vi "SAE J-1939 Gaslist add Signal Comments.vi"(10 "FTIR 1 Index":i32[](array[numeric])) -> (2 "FTIR 1 Name out":T1[](array[typedef]))   [LabVIEW 2020, in "CAN Konfig.lvlib"]
uses:
  CAN Konfig.lvlib
  Visualisierungs Elemente/String - Ausgabefeld.ctl
  FT-IR/FGV FT-IR Gasliste Aktionen.ctl
  <vilib>/regexp/Match Regular Expression.xnode
  FT-IR/FT-IR.lvlib
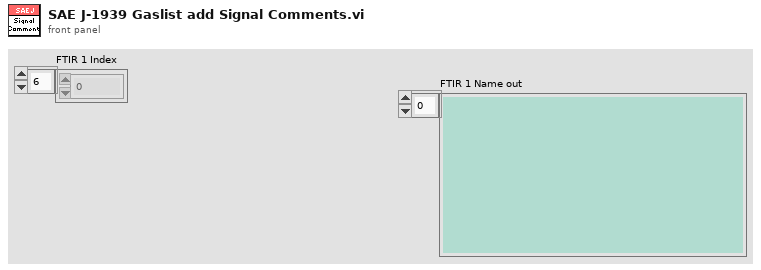
[diagram p1: front panel]
types:
  T1 = typedef "String - Ausgabefeld.ctl" = string
  T2 = typedef "FT-IR.lvlib/FGV FT-IR Gasliste Aktionen.ctl" = enum16{"lesen", "Gasliste FT-IR", "Gasliste ausgelesen", "laden", "speichern", "löschen"}
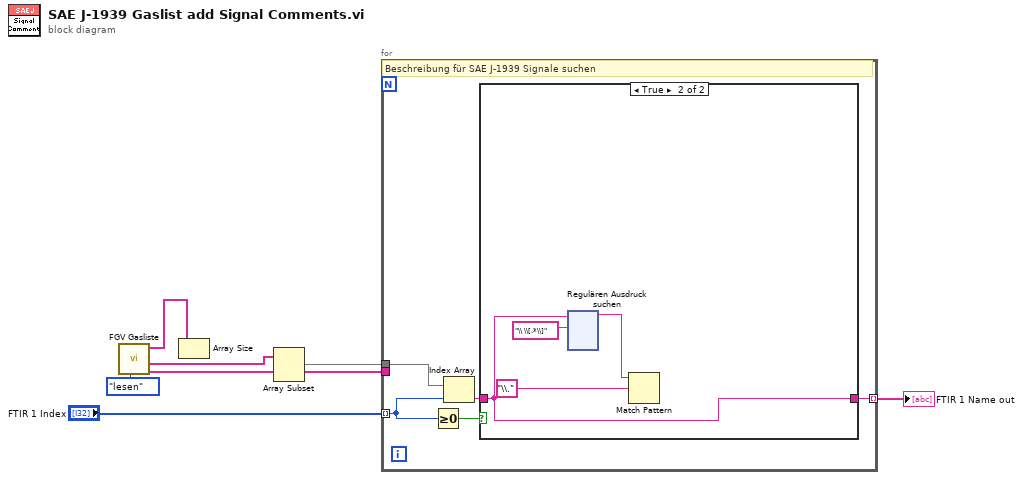
[diagram p0: block diagram]
diagram:
  n1 = call "FGV Gasliste.vi"("Aktionen"=FGV_FT-IR_Gasliste_Aktionen."lesen") -> ("Gasliste ausgelesen"=w2:T1[], "Aktuelle Gasliste gesamt"=w4:T1[], "Aktuelle Gasliste FT-IR"=w1:T1[])  [unwired: 8 in]
  n2 = Array Size(array=w1) -> ()  [unwired: 1 out]
  n3 = Array Subset(array=w4) -> (w6:T1[])  [unwired: 2 in]
  n4 = for {
    tunnel: "FTIR 1 Index" -> [w11] mode=indexing
    tunnel: w6 -> [w10]
    tunnel: [w8] -> w7 mode=indexing
    tunnel: w2 -> [_]
    # "Beschreibung für SAE J-1939 Signale suchen"
    n5 = Greater Or Equal To 0?(x=w11) -> (x >= 0?=w12:bool)
    n6 = Index Array(array=w10, index=w11) -> (element=w9:T1)
    n7 = case shown="True" w12 {
      tunnel: w9 -> [w13 w14]
      tunnel: [w13 w14] -> w8
      frame False {
      }
      frame True {
        n8 = xnode "Regulären Ausdruck suchen"("Eingangs-String"=w14, "Regulärer Ausdruck"="\\ \\[.*\\]") -> ("Vor Übereinstimmung"=w15:string)  [unwired: 4 in, 4 out]
        n9 = Match Pattern(string=w15, regular expression="\\." ("Such-String/-Zeichen (-)")) -> ()  [unwired: 1 in, 4 out]
      }
    }
  }
  "FTIR 1 Name out" <- w7
